vi "E1A_SOF Check.vi"(11 "Bytes data in":u8[](array[numeric])) -> (1 "Numeric":i32, 2 "Passed samples":i32, 3 "index of passed smpl":i32[](array[numeric]))   [LabVIEW 2022 SP3]
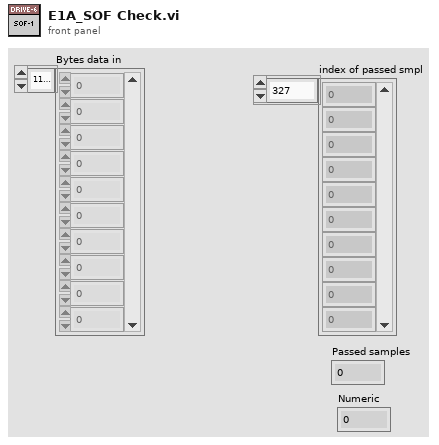
[diagram p1: front panel]
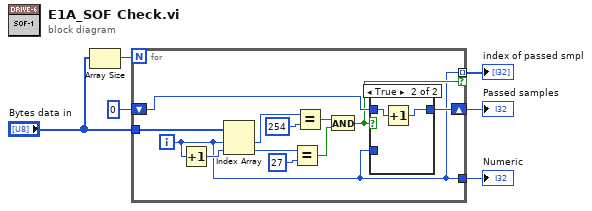
[diagram p0: block diagram]
diagram:
  n1 = Array Size(array="Bytes data in") -> (size(s)=w1:i32)
  n2 = for {
    N: w1 -> [_]
    tunnel: "Bytes data in" -> [w18]
    shift-right: [w9] -> w3
    shift-left: 0 ("x") -> [w10]
    tunnel: [w7] -> w4 mode=indexing if=w8
    tunnel: [w7] -> w5
    i -> [w7]
    n3 = Increment(x=w7) -> (x+1=w17:i32)
    n4 = Index Array(array=w18, index #1=w7, index #2=w17) -> (element #1=w16:u8, element #2=w14:u8)
    n5 = Equal?(x=w14, y=u8 27) -> (x = y?=w11:bool)
    n6 = Equal?(x=w16, y=u8 254) -> (x = y?=w12:bool)
    n7 = And(x=w12, y=w11) -> (x .and. y?=w8:bool)
    n8 = case shown="True" w8 {
      tunnel: w7 -> [_ _]
      tunnel: w10 -> [w19 w21]
      tunnel: [w19 w20] -> w9
      frame False {
      }
      frame True {
        n9 = Increment(x=w21) -> (x+1=w20:i32)
      }
    }
  }
  "Numeric" <- w5
  "index of passed smpl" <- w4
  "Passed samples" <- w3
